vi "SO-FSRS Analysis 2.0.vi"() -> ()   [LabVIEW 2014]
uses:
  <vilib>/Utility/file.llb/Read Delimited Spreadsheet (DBL).vi
  <vilib>/Math Plots/3D Math Plots/3D Surface/3D Surface Datatype/3D Surface Datatype.lvclass
  <vilib>/Math Plots/3D Math Plots/3D Scatter/3D Scatter Datatype/3D Scatter Datatype.lvclass
  <vilib>/gmath/NI_Gmath.lvlib
  <vilib>/Analysis/NI_AALPro.lvlib
  <vilib>/gmath/NumericalOptimization/LM model function reference.ctl
  <vilib>/gmath/NumericalOptimization/Nonlinear Curve Fit LM.vi
  <vilib>/Math Plots/3D Math Plots/3D Scatter/3D Scatter Datatype/Public/Plot Helper (Vector).vi
  <vilib>/Utility/file.llb/Write Delimited Spreadsheet (DBL).vi
  <vilib>/Math Plots/3D Math Plots/3D Scatter/3D Scatter Datatype/Public/Plot Helper (Matrix).vi
  <vilib>/Math Plots/3D Math Plots/3D Surface/3D Surface Datatype/Public/Plot Helper (Vector).vi
  <vilib>/Math Plots/3D Math Plots/3D Surface/3D Surface XCtrl/3D Surface.xctl
  LabView vis/Control 1.ctl
  LabView vis/Control 3.ctl
  <vilib>/Math Plots/3D Math Plots/3D Scatter/3D Scatter XCtrl/3D Scatter.xctl
panel:
  out "Shiftx":T1=[-400.0, -600.0, -200.0, -2100.0, -10.0, 570.0, 1700.0, 980.0, 10000.0, -1100.0, 150.0, 320.0, -850.0, -1500.0, -5000.0]
  in  "Load shiftx":bool
  in  "error in":errorcluster
  out "error out":errorcluster
  in  "Main Tab":T2(tab)
  in  "Shorter Name":string
  in  "Do it?":bool
  in  "Index":i32
  in  "What you gonna do":u16(ring) items=["Delete", "Flip"]
  in  "Folder - Batch Files":path
  out "Built Arrays":dbl[][](graph)
  in  "?":bool
  in  "File Names":u16(ring) items=["C", "D", "E"]
  out "Raw Data":dbl[][](graph)
  in  "List of Files":i32(listbox)
  in  "Batch 'em":bool
  in  "Load the batch":bool
  in  "List of Batch Files":i32(listbox)
  in  "Initial Vx":dbl
  in  "Final Vx":dbl
  in  "x rows":dbl
  in  "Initial Vy":dbl
  in  "Final Vy":dbl
  in  "y columns":dbl
  out "X Array (mV)":dbl[](array[numeric])
  out "Y Array (mV)":dbl[](array[numeric])
  in  "File Name":string
  in  "No. of Sets":i32
  in  "No. of Gr":i32
  in  "Flip?":bool
  out "String 2":string
  out "String":string
  out "Averaged Graph":cluster{"Shiftx":dbl[], "first row":dbl[]}(graph)
  in  "Load Sub":bool
  in  "List of Substracted Files":i32(listbox)
  in  "Folder - Substracted":path
  in  "Folder - Averaged":path
  in  "List of Averaged Files":i32(listbox)
  in  "?":bool
  in  "Subtract":bool
  in  "Average":bool
  out "Substracted Graph":cluster{"Value":dbl[], "first row":dbl[]}(graph)
  in  "Folder - TA":path
  in  "TA":bool
  out "Intensity Graph":dbl[][](graph)
  in  "Save Matrix?":bool
  out "3D Scatter":refnum<class "3D Plot Datatype.lvclass">[](xcontrol)
  in  "Time point":u16(ring) items=["-5000", "-1000", "-500", "0", "500", "1000", "2000", "3000", "4000", "5000", "6000", "7000", "8000", "9000", "10000", "15000", "20000", "25000", "30000", "35000", "40000", "45000", "50000", "60000", "70000", "80000", "90000", "100000", "120000", "140000", "160000", "180000", "200000", "220000", "240000", "260000", "280000", "300000", "320000", "340000", "360000", "380000", "400000", "420000", "440000", "460000", "480000", "500000"]
  out "3D Surface":refnum<class "3D Plot Datatype.lvclass">[](xcontrol)
  out "Raman Shift":dbl
  in  "Position Number (From 0 to 1328)":i32
  in  "You may begin":bool
  in  "Curve Fitting Time":bool
  in  "Curve Fitting\nOptions":enum32{"Batch", "XY Graphs", "XYZ Graphs"}(tab)
  in  "Batch Options":enum16{""}(ring)
  in  "XY Graph File":path
  in  "X axis":enum32{"shiftx", "times"}(radio)
  in  "Choose":enum32{"Standard Functions", "Custom Functions"}(radio)
  in  "Fitting method":u16(ring) items=["Least Square", "Least Absolute Residual", "Bisquare"]
  in  "Order":i32=2
  in  "Models":T3(radio)
  out "Equation of fit":string
  out "XY Graph":T4(graph)
  in  "Display Precision":i32=3 min=0
  out "Weighted Mean Square Error":dbl format="%#.3g"
  out "error information":string
  out "Fitted Y Values":dbl[](array[numeric]) format="%#.6g"
  in  "XYZ Graph File":path
  out "XYZ Fit Scatter":refnum<class "3D Plot Datatype.lvclass">[](xcontrol)
  in  "Vy Values":u16(ring) items=["-699", "-694", "-690", "-685", "-680", "-675", "-670"]
  in  "Vx Values":u16(ring) items=["-15", "-10", "-5", "0", "5", "10", "15"]
  in  "Time Delay":u16(ring) items=["-5000", "-1000", "-500", "0", "500", "1000", "2000", "3000", "4000", "5000", "6000", "7000", "8000", "9000", "10000", "15000", "20000", "25000", "30000", "35000", "40000", "45000", "50000", "60000", "70000", "80000", "90000", "100000", "120000", "140000", "160000", "180000", "200000", "220000", "240000", "260000", "280000", "300000", "320000", "340000", "360000", "380000", "400000", "420000", "440000", "460000", "480000", "500000"]
  in  "?":bool
  in  "Time points":T1=[-400.0, -600.0, -200.0, -2100.0, -10.0, 570.0, 1700.0, 980.0, 10000.0, -1100.0, 150.0, 320.0, -850.0, -1500.0, -5000.0]
  in  "Load":bool
  in  "Main Folder":T5
  # "Raster Scan Parameters"
  # "The first 2 distinct features you see are the probe spectrum \nwith the Raman pump on and off.\nThe Raman gain is shown too, but its amplitude is so \nmuch smaller it almost seems like it does not exist."
  # "Currently, this is linked to the Subtracted Folder. You can change it if that's not what you want."
  # "What I want on this page -  An X cross section, An Y cross section\n   I can move cursor to choose time and wavenumber  and checkfit\n\nWant a subset...Make a list of equations and fitting parameters fit wrt to timepoints, + x n y values....then,  plot what was plotted over there."
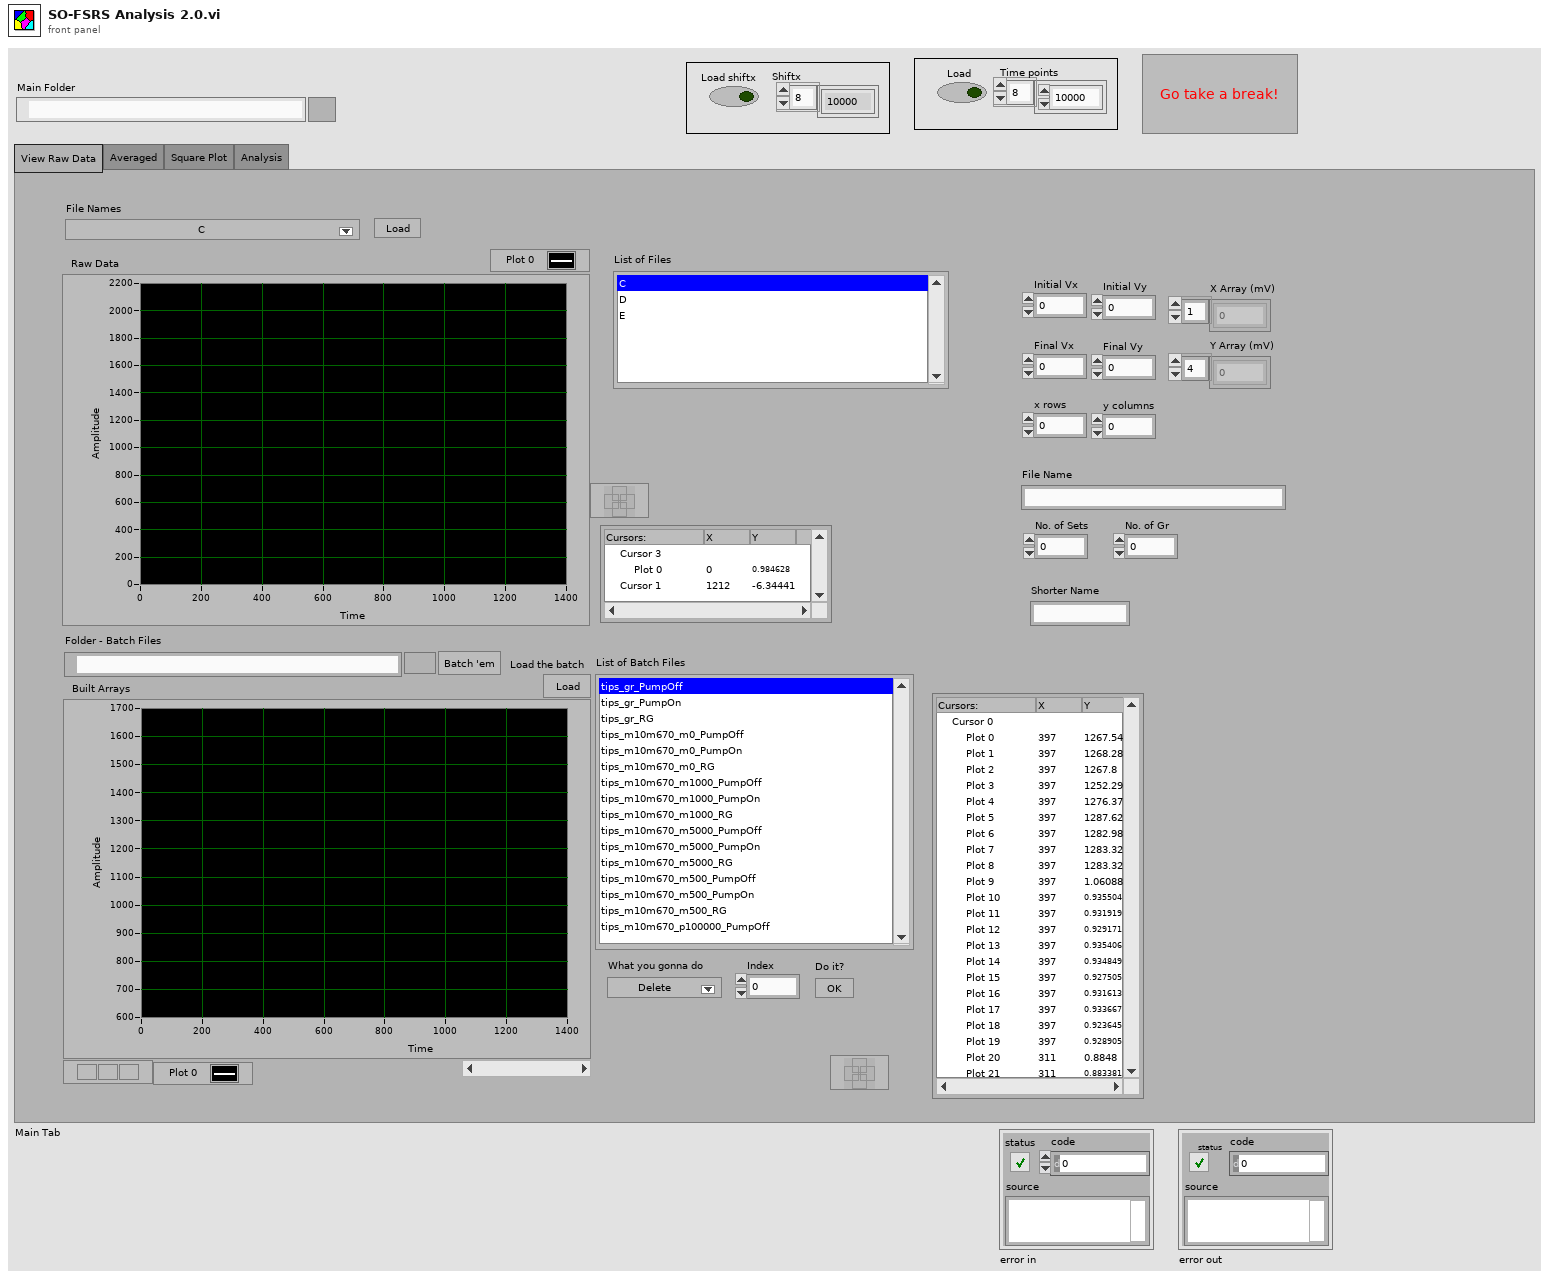
[diagram p1: front panel]
types:
  T1 = typedef "Control 3.ctl" = dbl[]
  T2 = enum32{"View Raw Data", "Averaged", "Square Plot", "Analysis"}
  T3 = enum32{"Linear", "Polynomial", "Exponential", "Power"}
  T4 = cluster{"Data":dbl[], "Best Exponential Fit":dbl[]}[]
  T5 = typedef "Control 1.ctl" = path
  T6 = typedef "NI_Gmath.lvlib/LM model function reference.ctl" = refnum<vi>
  T7 = cluster{"best nonlinear fit":dbl[], "best fit parameters":dbl[]}
  T8 = cluster{"best nonlinear fit":dbl[], "best fit parameters":dbl[]}[]
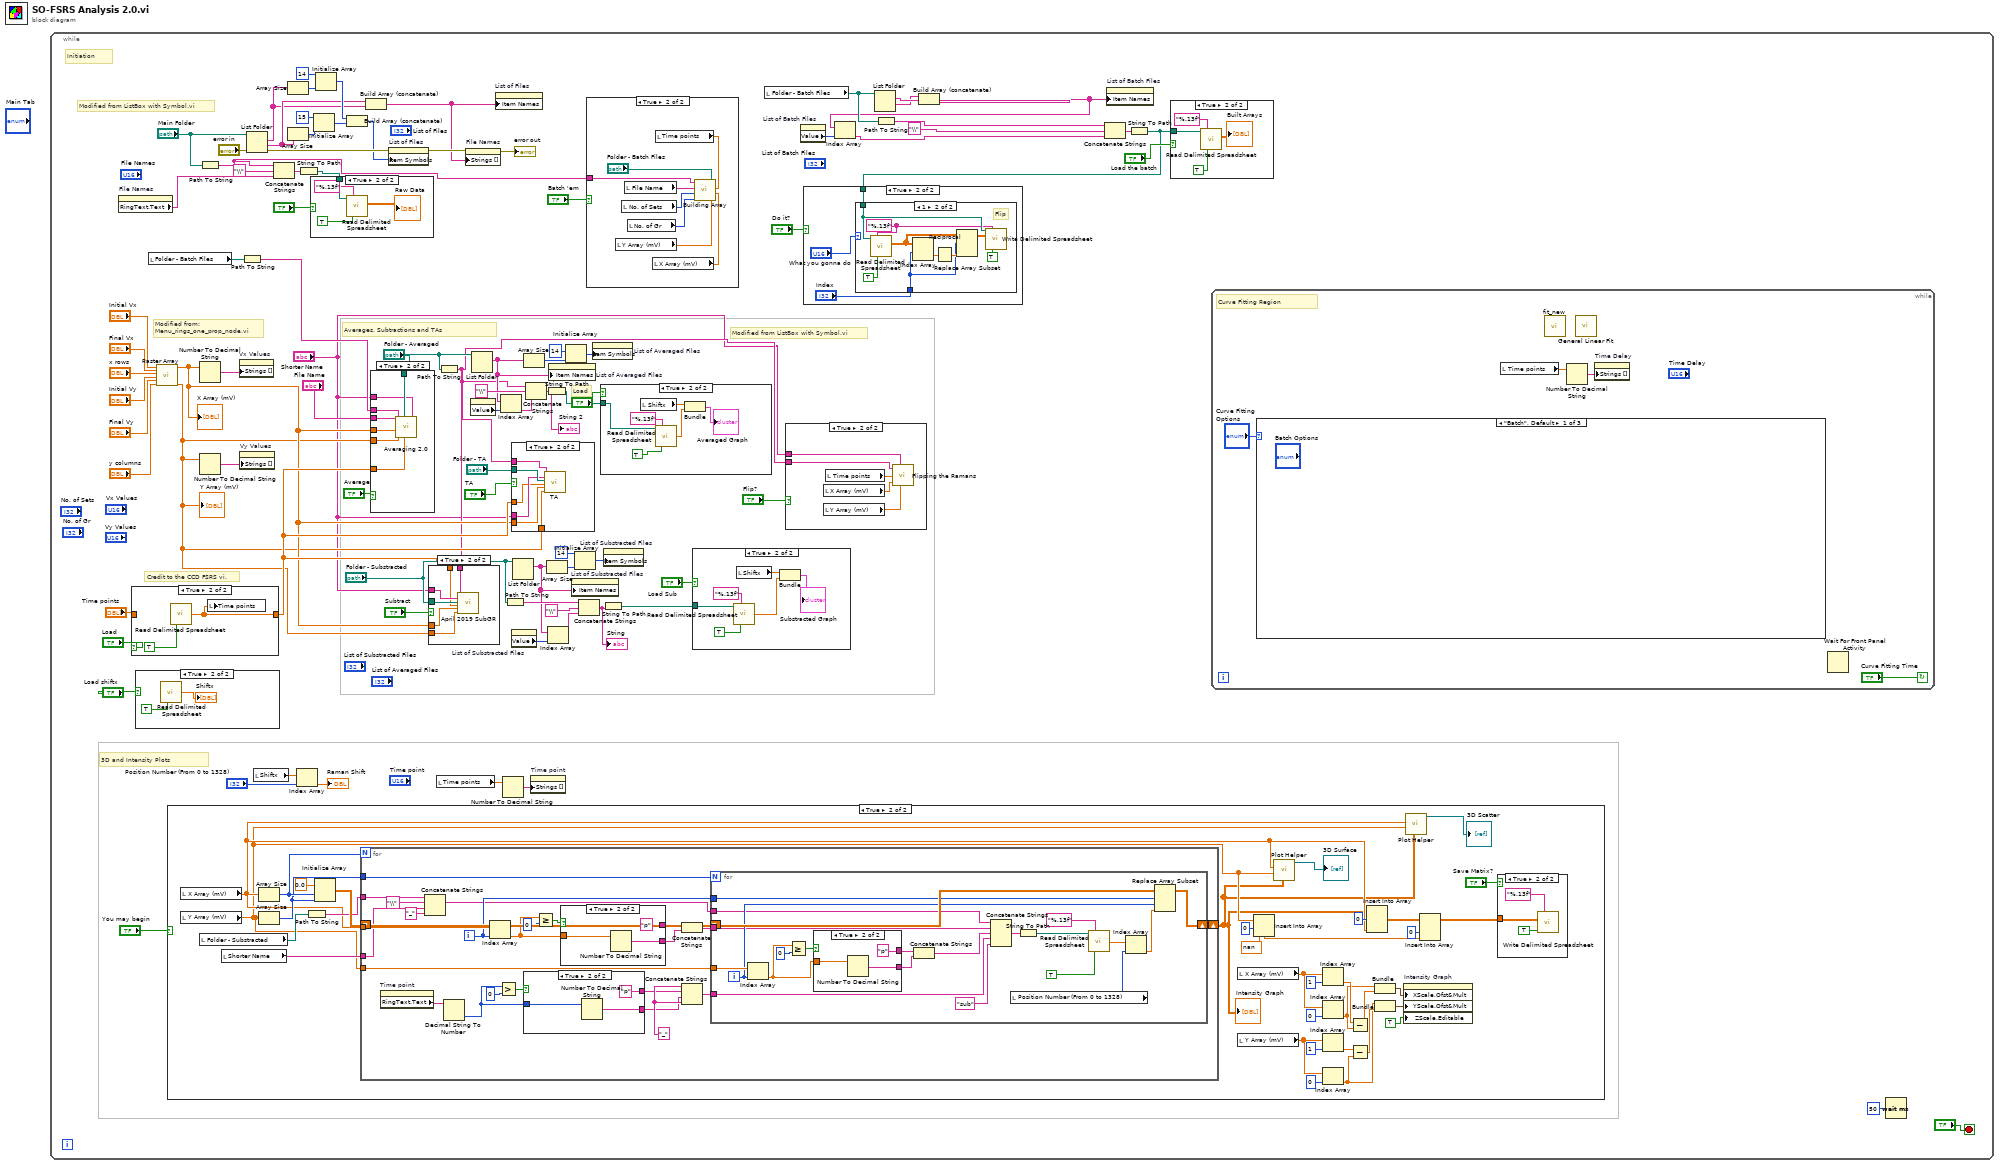
[diagram p0: block diagram]
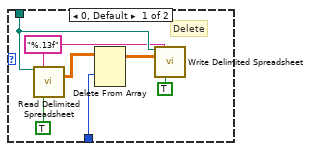
[diagram p5: hidden frame]
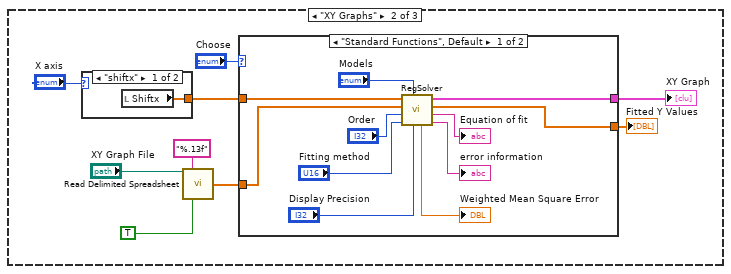
[diagram p9: hidden frame]
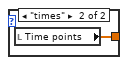
[diagram p10: hidden frame]
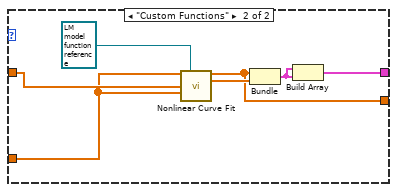
[diagram p11: hidden frame]
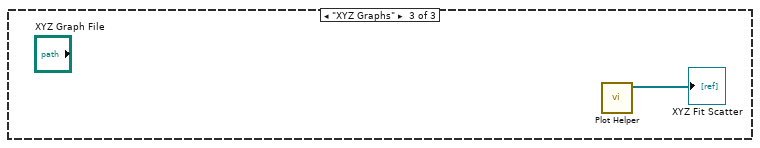
[diagram p12: hidden frame]
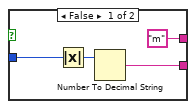
[diagram p15: hidden frame]
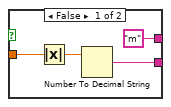
[diagram p16: hidden frame]
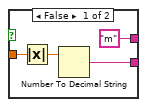
[diagram p17: hidden frame]
diagram:
  n1 = while {
    stop <- "?" stop-if-true
    # "Load"
    # "Initiation"
    # "3D and Intensity Plots"
    # "Averages, Subtractions and TAs"
    # "Modified from:\nMenu_rings_one_prop_node.vi"
    # "Modified from ListBox with Symbol.vi"
    # "Credit to the CCD FSRS vi."
    # "Modified from ListBox with Symbol.vi"
    n2 = property on="File Names" class="Ring (strict)"() -> ("RingText.Text"=w69:string)  [unwired: 2 in, 2 out]
    n3 = case shown="True" "Load" {
      tunnel: [w303 w304] -> w10
      tunnel: "Time points" -> [w303 _]
      frame False {
      }
      frame True {
        n4 = call-poly <vilib>:"Read Delimited Spreadsheet.vi"("transpose? (F)"=TRUE ("transpose (no:F)")) -> ("first row"=w304:dbl[])  [unwired: 9 in, 5 out]
        n5 = local write "Time points"(w304) -> ()
      }
    }
    n6 = case shown="True" "Load shiftx" {
      frame False {
      }
      frame True {
        n7 = call-poly <vilib>:"Read Delimited Spreadsheet.vi"("transpose? (F)"=TRUE) -> ("first row"=→"Shiftx":dbl[])  [unwired: 9 in, 5 out]
      }
    }
    n8 = local read "Folder - Batch Files"() -> (w14:path)
    n9 = call "Raster Array.vi"("Initial Vx"="Initial Vx", "Final Vx"="Final Vx", "x rows"="x rows", "Initial Vy"="Initial Vy", "Final Vy"="Final Vy", "y columns"="y columns") -> ("X Array"=w9:dbl[], "Y Array"=w8:dbl[])  [unwired: 12 in]
    "X Array (mV)" <- w9
    "Y Array (mV)" <- w8
    n10 = case shown="True" "You may begin" {
      frame False {
      }
      frame True {
        n11 = local read "X Array (mV)"() -> (w173:dbl[])
        n12 = local read "Y Array (mV)"() -> (w172:dbl[])
        n13 = local read "Folder - Substracted"() -> (w199:path)
        n14 = local read "Shorter Name"() -> (w197:string)
        n15 = Array Size(array=w173) -> (size(s)=w196:i32)
        n16 = Array Size(array=w172) -> (size(s)=w195:i32)
        n17 = Path To String(path=w199) -> (string=w198:string)
        n18 = Initialize Array(0.0 ("element"), w196, w195) -> (w200:dbl[][])
        n19 = for {
          N: w196 -> [_]
          shift-right: [w229] -> w168
          shift-left: w200 -> [w230]
          tunnel: w173 -> [w226]
          tunnel: w172 -> [w223]
          tunnel: w198 -> [w222]
          tunnel: w197 -> [w221]
          tunnel: w195 -> [w208]
          i -> [w225]
          w214 = "_" ("string")
          n20 = property on="Time point" class="Ring (strict)"() -> ("RingText.Text"=w207:string)  [unwired: 2 in, 2 out]
          n21 = Concatenate Strings(w222, "\\", w221, "_" ("string")) -> (w216:string)
          n22 = Decimal String To Number(string=w207) -> (number=w206:i32)  [unwired: 2 in, 1 out]
          n23 = Index Array(array=w226, index=w225) -> (element=w224:dbl)
          n24 = Greater?(x=w206, y=0) -> (0:w212:bool)
          n25 = case shown="True" w212 {
            tunnel: ["m" "p"] -> w211
            tunnel: w206 -> [w233 w236]
            tunnel: [w231 w235] -> w210
            frame False {
              n26 = Absolute Value(x=w233) -> (abs(x)=w232:i32)
              n27 = Number To Decimal String(number=w232) -> (decimal integer string=w231:string)  [unwired: 1 in]
            }
            frame True {
              n28 = Number To Decimal String(number=w236) -> (decimal integer string=w235:string)  [unwired: 1 in]
            }
          }
          n29 = Greater Or Equal?(x=w224, y=0) -> (x >= y?=w228:bool)
          n30 = case shown="True" w228 {
            tunnel: ["m" "p"] -> w218
            tunnel: w224 -> [w240 w242]
            tunnel: [w238 w243] -> w217
            frame False {
              n31 = Absolute Value(x=w240) -> (abs(x)=w239:dbl)
              n32 = Number To Decimal String(number=w239) -> (decimal integer string=w238:string)  [unwired: 1 in]
            }
            frame True {
              n33 = Number To Decimal String(number=w242) -> (decimal integer string=w243:string)  [unwired: 1 in]
            }
          }
          n34 = Concatenate Strings(w218, w217) -> (w215:string)
          n35 = Concatenate Strings(w214, w211, w210, w214) -> (w209:string)
          n36 = for {
            N: w208 -> [_]
            shift-right: [w265] -> w229
            shift-left: w230 -> [w266]
            tunnel: w225 -> [w264]
            tunnel: w223 -> [w261]
            tunnel: w216 -> [w256]
            tunnel: w215 -> [w255]
            tunnel: w209 -> [w252]
            i -> [w260]
            n37 = Index Array(array=w261, index=w260) -> (element=w259:dbl)
            n38 = Greater Or Equal?(x=w259, y=0) -> (x >= y?=w263:bool)
            n39 = case shown="True" w263 {
              tunnel: ["m" "p"] -> w258
              tunnel: w259 -> [w269 w271]
              tunnel: [w267 w272] -> w257
              frame False {
                n40 = Absolute Value(x=w269) -> (abs(x)=w268:dbl)
                n41 = Number To Decimal String(number=w268) -> (decimal integer string=w267:string)  [unwired: 1 in]
              }
              frame True {
                n42 = Number To Decimal String(number=w271) -> (decimal integer string=w272:string)  [unwired: 1 in]
              }
            }
            n43 = Concatenate Strings(w258, w257) -> (w254:string)
            n44 = Concatenate Strings(w256, w255, w254, w252, "sub" ("string")) -> (w245:string)
            n45 = local read "Position Number (From 0 to 1328)"() -> (w247:i32)
            n46 = String To Path(string=w245) -> (path=w251:path)
            n47 = call-poly <vilib>:"Read Delimited Spreadsheet.vi"("file path (dialog if empty)"=w251, "format (%.3f)"="%.13f", "transpose? (F)"=TRUE) -> ("first row"=w248:dbl[])  [unwired: 7 in, 5 out]
            n48 = Index Array(array=w248, index=w247) -> (element=w246:dbl)
            n49 = Replace Array Subset(array=w266, new element=w246, index (row)=w264, index (col)=w260) -> (w265:dbl[][])
          }
        }
        "Intensity Graph" <- w168
        n50 = local read "X Array (mV)"() -> (w194:dbl[])
        n51 = local read "Y Array (mV)"() -> (w188:dbl[])
        n52 = Insert Into Array(array=w172, index=0, new element=nan ("new element/subarray")) -> (w169:dbl[])
        n53 = call-poly <vilib>:"Plot Helper.vi"("z matrix"=w168, "y vector"=w172, "x vector"=w173) -> ("3D Plot lvclass Array out"=→"3D Surface":refnum<class "3D Plot Datatype.lvclass">[])  [unwired: 3 in, 5 out]
        n54 = Index Array(array=w194, index=1) -> (element=w191:dbl)
        n55 = Index Array(array=w194, index=0) -> (element=w189:dbl)
        n56 = Index Array(array=w188, index=1) -> (element=w184:dbl)
        n57 = Index Array(array=w188, index=0) -> (element=w183:dbl)
        n58 = Subtract(x=w191, y=w189) -> (x-y=w190:dbl)
        n59 = Subtract(x=w184, y=w183) -> (x-y=w185:dbl)
        n60 = Insert Into Array(array=w168, index (row)=0, new element=w173) -> (w177:dbl[][])  [unwired: 1 in]
        n61 = Bundle("Numeric"=w189, w190) -> (w181:cluster{"Numeric":dbl, dbl})  [unwired: 1 in]
        n62 = Bundle("Numeric"=w183, w185) -> (w180:cluster{"Numeric":dbl, dbl})  [unwired: 1 in]
        n63 = property on="Intensity Graph" class="IntGraph (strict)"("XScale.Ofst&Mult"=w181, "YScale.Ofst&Mult"=w180, "ZScale.Editable"=TRUE ("Z Scale.Editable")) -> ()  [unwired: 2 in, 2 out]
        n64 = call-poly <vilib>:"Plot Helper.vi"("z matrix"=w168, "y vector"=w172, "x vector"=w173) -> ("3D Plot lvclass Array out"=→"3D Scatter":refnum<class "3D Plot Datatype.lvclass">[])  [unwired: 3 in, 5 out]
        n65 = Insert Into Array(array=w177, index (col)=0 ("disabled index (col)"), new element=w169) -> (w176:dbl[][])  [unwired: 1 in]
        n66 = case shown="True" "Save Matrix?" {
          tunnel: w176 -> [_ w203]
          frame False {
          }
          frame True {
            n67 = call-poly <vilib>:"Write Delimited Spreadsheet.vi"("format (%.3f)"="%.13f", "2D data"=w203, "transpose? (F)"=TRUE) -> ()  [unwired: 11 in, 2 out]
          }
        }
      }
    }
    n68 = Number To Decimal String(number=w9) -> (decimal integer string=w53:string[])  [unwired: 1 in]
    n69 = Number To Decimal String(number=w8) -> (decimal integer string=w52:string[])  [unwired: 1 in]
    n70 = Path To String(path="Main Folder") -> (string=w34:string)
    n71 = property on="Vx Values" class="Ring (strict)"("Strings []"=w53) -> ()  [unwired: 2 in, 2 out]
    n72 = property on="Vy Values" class="Ring (strict)"("Strings []"=w52) -> ()  [unwired: 2 in, 2 out]
    n73 = Path To String(path=w14) -> (string=w15:string)
    n74 = List Folder(path="Main Folder", error in="error in") -> (filenames=w76:string[], folder names=w80:string[], error out=w84:errorcluster)  [unwired: 2 in, 1 out]
    n75 = local read "Shiftx"() -> (w38:T1)
    n76 = Concatenate Strings(w34, "\\", w69) -> (w74:string)
    n77 = Array Size(array=w80) -> (size(s)=w78:i32)
    n78 = Array Size(array=w76) -> (size(s)=w77:i32)
    n79 = Index Array(array=w38, index="Position Number (From 0 to 1328)") -> (element=→"Raman Shift":dbl)
    n80 = String To Path(string=w74) -> (path=w73:path)
    n81 = case shown="True" "?" {
      tunnel: w73 -> [_ w302]
      frame False {
      }
      frame True {
        n82 = call-poly <vilib>:"Read Delimited Spreadsheet.vi"("file path (dialog if empty)"=w302, "format (%.3f)"="%.13f", "transpose? (F)"=TRUE) -> ("all rows"=→"Raw Data":dbl[][])  [unwired: 7 in, 5 out]
      }
    }
    n83 = Initialize Array(15 ("Numeric"), w78) -> (w82:i32[])
    n84 = Initialize Array(14 ("Numeric 2"), w77) -> (w81:i32[])
    n85 = Build Array (concatenate)(w81, w82) -> (w83:i32[])
    n86 = Build Array (concatenate)(w80, w76) -> (w61:string[])
    n87 = case shown="True" "Average" {
      tunnel: "File Name" -> [_ w298]
      tunnel: w15 -> [_ w297]
      tunnel: w10 -> [_ w295]
      tunnel: w9 -> [_ w293]
      tunnel: w8 -> [_ w294]
      tunnel: "Folder - Averaged" -> [_ w296]
      tunnel: "Shorter Name" -> [_ w292]
      frame False {
      }
      frame True {
        n88 = call "Averaging 2.0.vi"("Shorter Name"=w292, "Timepoints"=w295, "Folder to Save"=w296, "Vy array"=w294, "Vx array"=w293, "Name of File"=w298, "Folder Name"=w297) -> ()
      }
    }
    n89 = property on="List of Files" class="LstBox (strict)"(error in=w84, "Item Symbols"=w83) -> (error out=w71:errorcluster)  [unwired: 1 in, 1 out]
    n90 = local read "Time points"() -> (w41:T1)
    n91 = Path To String(path="Folder - Averaged") -> (string=w4:string)
    n92 = case shown="True" "Subtract" {
      tunnel: "Folder - Substracted" -> [_ w285]
      tunnel: w4 -> [_ w284]
      tunnel: "Shorter Name" -> [_ w283]
      tunnel: w10 -> [_ w282]
      tunnel: w9 -> [_ w281]
      tunnel: w8 -> [_ w280]
      frame False {
      }
      frame True {
        n93 = call "April 2019 SubGR.vi"("Folder Name"=w284, "Name of File"=w283, "Folder to Save"=w285, "Timepoints"=w282, "Vx array"=w281, "Vy array"=w280) -> ()  [unwired: 14 in]
      }
    }
    n94 = property on="File Names" class="Ring (strict)"(error in=w71, "Strings []"=w61) -> (error out=→"error out":errorcluster)  [unwired: 1 in, 1 out]
    n95 = property on="List of Averaged Files" class="LstBox (strict)"() -> ("Value"=w20:i32)  [unwired: 2 in, 2 out]
    n96 = List Folder(path="Folder - Averaged") -> (filenames=w21:string[])  [unwired: 3 in, 3 out]
    n97 = property on="List of Files" class="LstBox (strict)"("Item Names"=w61) -> ()  [unwired: 2 in, 2 out]
    n98 = Index Array(array=w21, index=w20) -> (element=w19:string)
    n99 = Number To Decimal String(number=w41) -> (decimal integer string=w42:string[])  [unwired: 1 in]
    n100 = Path To String(path="Folder - Substracted") -> (string=w45:string)
    n101 = case shown="True" "TA" {
      tunnel: "Folder - TA" -> [_ w100]
      tunnel: "Shorter Name" -> [_ w99]
      tunnel: w4 -> [_ w98]
      tunnel: w10 -> [_ w97]
      tunnel: w9 -> [_ w96]
      tunnel: w8 -> [_ w95]
      frame False {
      }
      frame True {
        n102 = call "TA.vi"("Folder Name"=w98, "Name of File"=w99, "Folder to Save"=w100, "Timepoints"=w97, "Vx array"=w96, "Vy array"=w95) -> ()  [unwired: 14 in]
      }
    }
    n103 = property on="List of Substracted Files" class="LstBox (strict)"() -> ("Value"=w18:i32)  [unwired: 2 in, 2 out]
    n104 = List Folder(path="Folder - Substracted") -> (filenames=w17:string[])  [unwired: 3 in, 3 out]
    n105 = Array Size(array=w21) -> (size(s)=w66:i32)
    n106 = Concatenate Strings(w4, "\\", w19) -> (w6:string)
    "String 2" <- w6
    n107 = property on="Time point" class="Ring (strict)"("Strings []"=w42) -> ()  [unwired: 2 in, 2 out]
    n108 = String To Path(string=w6) -> (path=w64:path)
    n109 = Array Size(array=w17) -> (size(s)=w50:i32)
    n110 = Index Array(array=w17, index=w18) -> (element=w16:string)
    n111 = property on="List of Averaged Files" class="LstBox (strict)"("Item Names"=w21) -> ()  [unwired: 2 in, 2 out]
    n112 = Initialize Array(14 ("Numeric 2"), w66) -> (w67:i32[])
    n113 = property on="List of Substracted Files" class="LstBox (strict)"("Item Names"=w17) -> ()  [unwired: 2 in, 2 out]
    n114 = Initialize Array(14 ("Numeric 2"), w50) -> (w48:i32[])
    n115 = Concatenate Strings(w45, "\\", w16) -> (w5:string)
    "String" <- w5
    n116 = case shown="True" "Batch 'em" {
      tunnel: w34 -> [_ w131]
      frame False {
      }
      frame True {
        n117 = local read "Y Array (mV)"() -> (w126:dbl[])
        n118 = local read "No. of Sets"() -> (w125:i32)
        n119 = local read "File Name"() -> (w130:string)
        n120 = local read "No. of Gr"() -> (w124:i32)
        n121 = local read "X Array (mV)"() -> (w127:dbl[])
        n122 = local read "Time points"() -> (w128:T1)
        n123 = call "Building Array.vi"("Vy array"=w126, "Vx array"=w127, "Timepoints"=w128, "Folder to Save"="Folder - Batch Files", "No. of Gr"=w124, "No. of Sets"=w125, "Name of File"=w130, "Folder Name"=w131) -> ()
      }
    }
    n124 = property on="List of Averaged Files" class="LstBox (strict)"("Item Symbols"=w67) -> ()  [unwired: 2 in, 2 out]
    n125 = case shown="True" "?" {
      tunnel: w64 -> [_ w291]
      frame False {
      }
      frame True {
        n126 = local read "Shiftx"() -> (w287:T1)
        n127 = call-poly <vilib>:"Read Delimited Spreadsheet.vi"("file path (dialog if empty)"=w291, "format (%.3f)"="%.13f", "transpose? (F)"=TRUE) -> ("first row"=w286:dbl[])  [unwired: 7 in, 5 out]
        n128 = Bundle("Shiftx"=w287, "first row"=w286) -> (→"Averaged Graph":cluster{"Shiftx":T1, "first row":dbl[]})  [unwired: 1 in]
      }
    }
    n129 = String To Path(string=w5) -> (path=w37:path)
    n130 = property on="List of Substracted Files" class="LstBox (strict)"("Item Symbols"=w48) -> ()  [unwired: 2 in, 2 out]
    n131 = case shown="True" "Load Sub" {
      tunnel: w37 -> [_ w279]
      frame False {
      }
      frame True {
        n132 = call-poly <vilib>:"Read Delimited Spreadsheet.vi"("file path (dialog if empty)"=w279, "format (%.3f)"="%.13f", "transpose? (F)"=TRUE) -> ("first row"=w276:dbl[])  [unwired: 7 in, 5 out]
        n133 = local read "Shiftx"() -> (w274:T1)
        n134 = Bundle("Shiftx"=w274, "first row"=w276) -> (→"Substracted Graph":cluster{"Shiftx":T1, "first row":dbl[]})  [unwired: 1 in]
      }
    }
    n135 = local read "Folder - Batch Files"() -> (w31:path)
    n136 = case shown="True" "Flip?" {
      tunnel: w4 -> [_ w94]
      tunnel: "Shorter Name" -> [_ w93]
      frame False {
      }
      frame True {
        n137 = local read "X Array (mV)"() -> (w91:dbl[])
        n138 = local read "Y Array (mV)"() -> (w90:dbl[])
        n139 = local read "Time points"() -> (w92:T1)
        n140 = call "Flipping the Ramans.vi"("Folder Name"=w94, "Name of File"=w93, "Timepoints"=w92, "Vx array"=w91, "Vy array"=w90) -> ()  [unwired: 1 in]
      }
    }
    n141 = property on="List of Batch Files" class="LstBox (strict)"() -> ("Value"=w24:i32)  [unwired: 2 in, 2 out]
    n142 = List Folder(path=w31) -> (filenames=w27:string[], folder names=w1:string[])  [unwired: 3 in, 2 out]
    n143 = Path To String(path=w31) -> (string=w30:string)
    n144 = Build Array (concatenate)(w1, w27) -> (w23:string[])
    n145 = Index Array(array=w23, index=w24) -> (element=w22:string)
    n146 = Concatenate Strings(w30, "\\", w22) -> (w28:string)
    n147 = property on="List of Batch Files" class="LstBox (strict)"("Item Names"=w23) -> ()  [unwired: 2 in, 2 out]
    n148 = String To Path(string=w28) -> (path=w25:path)
    n149 = case shown="True" "Do it?" {
      tunnel: w25 -> [_ w102]
      frame False {
      }
      frame True {
        n150 = case shown="1" "What you gonna do" {
          tunnel: w102 -> [w106 w112]
          tunnel: "Index" -> [w108 w115]
          frame 0, Default {
            w105 = "%.13f" ("format (%.3f)")
            # "Delete"
            n151 = call-poly <vilib>:"Read Delimited Spreadsheet.vi"("file path (dialog if empty)"=w106, "format (%.3f)"=w105, "transpose? (F)"=TRUE) -> ("all rows"=w109:dbl[][])  [unwired: 7 in, 5 out]
            n152 = Delete From Array(array=w109, index (row)=w108) -> (array with subset deleted=w107:dbl[][])  [unwired: 2 in, 1 out]
            n153 = call-poly <vilib>:"Write Delimited Spreadsheet.vi"("file path (dialog if empty)"=w106, "format (%.3f)"=w105, "2D data"=w107, "transpose? (F)"=TRUE) -> ()  [unwired: 10 in, 2 out]
          }
          frame 1 {
            w111 = "%.13f" ("format (%.3f)")
            # "Flip"
            n154 = call-poly <vilib>:"Read Delimited Spreadsheet.vi"("file path (dialog if empty)"=w112, "format (%.3f)"=w111, "transpose? (F)"=TRUE) -> ("all rows"=w117:dbl[][])  [unwired: 7 in, 5 out]
            n155 = Index Array(array=w117, index (row)=w115) -> (element=w118:dbl[])  [unwired: 1 in]
            n156 = Reciprocal(x=w118) -> (1/x=w116:dbl[])
            n157 = Replace Array Subset(array=w117, new element=w116, index (row)=w115) -> (w113:dbl[][])  [unwired: 1 in]
            n158 = call-poly <vilib>:"Write Delimited Spreadsheet.vi"("file path (dialog if empty)"=w112, "format (%.3f)"=w111, "2D data"=w113, "transpose? (F)"=TRUE) -> ()  [unwired: 10 in, 2 out]
          }
        }
      }
    }
    n159 = case shown="True" "Load the batch" {
      tunnel: w25 -> [_ w120]
      frame False {
      }
      frame True {
        n160 = call-poly <vilib>:"Read Delimited Spreadsheet.vi"("file path (dialog if empty)"=w120, "format (%.3f)"="%.13f", "transpose? (F)"=TRUE) -> ("all rows"=→"Built Arrays":dbl[][])  [unwired: 7 in, 5 out]
      }
    }
    n161 = while {
      stop <- "Curve Fitting Time" continue-if-true
      # "Curve Fitting Region"
      n162 = case shown="\"Batch\", Default" "Curve Fitting\nOptions" {
        frame "Batch", Default {
        }
        frame "XY Graphs" {
          n163 = case shown="\"shiftx\"" "X axis" {
            tunnel: [w147 w148] -> w141
            frame "shiftx" {
              n164 = local read "Shiftx"() -> (w147:T1)
            }
            frame "times" {
              n165 = local read "Time points"() -> (w148:T1)
            }
          }
          n166 = call-poly <vilib>:"Read Delimited Spreadsheet.vi"("file path (dialog if empty)"="XY Graph File", "format (%.3f)"="%.13f", "transpose? (F)"=TRUE) -> ("first row"=w143:dbl[])  [unwired: 7 in, 5 out]
          n167 = case shown="\"Standard Functions\", Default" "Choose" {
            tunnel: [w153 w165] -> w139
            tunnel: [w152 w164] -> w140
            tunnel: w143 -> [w150 w160]
            tunnel: w141 -> [w149 w163]
            frame "Standard Functions", Default {
              n168 = call "RegSolver.vi"("Display Precision"="Display Precision", "Models"="Models", "Fitting method"="Fitting method", "Order"="Order", "Y Data"=w150, "X Data"=w149) -> ("error information"=→"error information":string, "Equation of fit"=→"Equation of fit":string, "Fitted Data"=w152:dbl[], "XY Graph"=w153:T4, "MSE"=→"Weighted Mean Square Error":dbl)  [unwired: 1 in]
            }
            frame "Custom Functions" {
              n169 = call-poly <vilib>:"Nonlinear Curve Fit.vi"("Y"=w160, "f(x,a)"=T6 refnum, "Weight"=w163, "initial parameters"=w160) -> ("best nonlinear fit"=w164:dbl[], "best fit parameters"=w166:dbl[])  [unwired: 6 in, 4 out]
              n170 = Bundle("best nonlinear fit"=w164, "best fit parameters"=w166) -> (w162:T7)  [unwired: 1 in]
              n171 = Build Array(w162, w162) -> (w165:T8)
            }
          }
          "Fitted Y Values" <- w140
          "XY Graph" <- w139
        }
        frame "XYZ Graphs" {
          n172 = call-poly <vilib>:"Plot Helper.vi"() -> ("3D Plot lvclass Array out"=→"XYZ Fit Scatter":refnum<class "3D Plot Datatype.lvclass">[])  [unwired: 6 in, 5 out]
        }
      }
      n173 = local read "Time points"() -> (w136:T1)
      n174 = call "fit_new.vi"() -> ()  [unwired: 10 in, 2 out]
      n175 = Number To Decimal String(number=w136) -> (decimal integer string=w137:string[])  [unwired: 1 in]
      n176 = call <vilib>:"General Linear Fit.vi"() -> ()  [unwired: 10 in, 6 out]
      n177 = property on="Time Delay" class="Ring (strict)"("Strings []"=w137) -> ()  [unwired: 2 in, 2 out]
      n178 = Wait For Front Panel Activity() -> ()  [unwired: 3 in, 1 out]
    }
    n179 = Wait (ms)(milliseconds to wait=u32 50) -> ()  [unwired: 1 out]
  }
